vi "Constructor.vi"(8 "error in":errorcluster, 10 "Id":string, 11 "Name":string) -> (0 "error out":errorcluster, 3 "SequenceRunReference out":refnum<class "SequenceRunReference.lvclass">)   [LabVIEW 2021, in "ProligentXMLGenerator.lvlib" / "SequenceRunReference.lvclass"]
uses:
  SequenceRunReference.lvclass
  SequenceRunReference.lvclass/SequenceRunReference.ctl
  Data.ctl
  Base/Guid/Guid.lvclass
  Model/CustomData/CustomData.lvclass
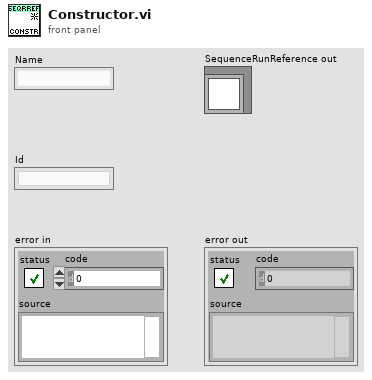
[diagram p1: front panel]
types:
  T1 = typedef "ProligentXMLGenerator.lvlib/SequenceRunReference.lvclass/Data.ctl" = cluster{"Name":string, "CustomData":refnum<class "CustomData.lvclass">, "Id":refnum<class "Guid.lvclass">}
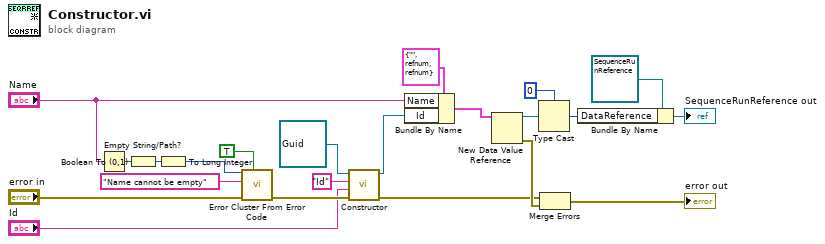
[diagram p0: block diagram]
diagram:
  n1 = Empty String/Path?(string/path="Name") -> (empty?=w11:bool)
  n2 = Boolean To (0,1)(Boolean=w11) -> (0, 1=w10:i16)
  n3 = To Long Integer(number=w10) -> (32bit integer=w9:i32)
  n4 = call <vilib>:"Error Cluster From Error Code.vi"("show call chain? (False)"=TRUE, "error in (no error)"="error in", "error message (\"\")"="Name cannot be empty" ("error message (\"\")"), "error code (0)"=w9) -> ("error out"=w4:errorcluster)  [unwired: 5 in]
  n5 = call-dynamic "Constructor.vi"("error in"=w4, "Value"="Id", "Name"="Id", "String in"=refnum<class "Guid.lvclass"> refnum ("ProligentCanonicalFile:Guid.lvclass")) -> ("error out"=w1:errorcluster, "String out"=w5:refnum<class "Guid.lvclass">)  [unwired: 6 in]
  n6 = Bundle By Name(cluster=T1 {"Name"="", "CustomData"=refnum, "Id"=refnum} ("Data"), "Name"="Name", "Id"=w5) -> (w18:T1)
  n7 = New Data Value Reference(data value=w18) -> (data value reference=w17:refnum<data-value>, error out=w14:errorcluster)  [unwired: 1 in]
  n8 = Type Cast(type=u64 0, x=w17) -> (*(type *) &x=w15:u64)
  n9 = Merge Errors(w1, w14) -> (→"error out":errorcluster)
  n10 = Bundle By Name(cluster=refnum<class "SequenceRunReference.lvclass"> refnum ("ProligentResultProcessor:Defect"), "DataReference"=w15) -> (→"SequenceRunReference out":refnum<class "SequenceRunReference.lvclass">)
